vi "private-TestableClass FirstTest.vi"(8 "error in (no error)":errorcluster, 11 "Caraya-TestableClass in":refnum<class "Caraya-TestableClass.lvclass">) -> (0 "error out":errorcluster)   [LabVIEW 2013, in "Caraya-TestableClass.lvclass"]
uses:
  Caraya-TestableClass.lvclass
  Caraya-TestableClass.lvclass/Caraya-TestableClass.ctl
  classes/Test/Test.lvclass
  classes/Assert/Assert.lvclass
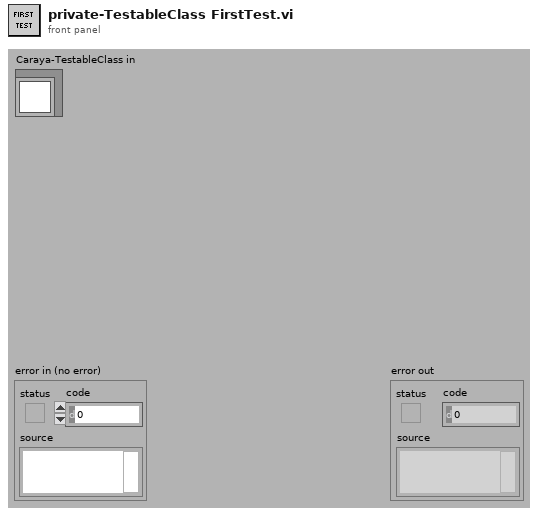
[diagram p1: front panel]
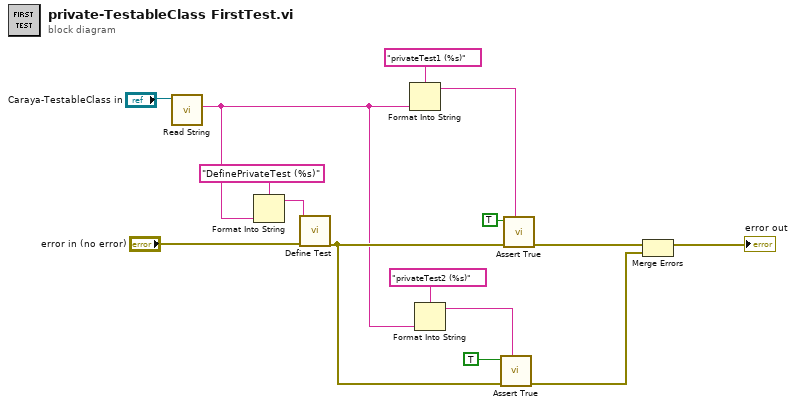
[diagram p0: block diagram]
diagram:
  n1 = call "Read String.vi"("Caraya-TestableClass in"="Caraya-TestableClass in") -> ("String"=w2:string)  [unwired: 9 in, 1 out]
  n2 = Format Into String(format string="DefinePrivateTest (%s)" ("Label (VI Title)"), w2) -> (resulting string=w8:string)  [unwired: 2 in, 1 out]
  n3 = call "Define Test.vi"("error in (no error)"="error in (no error)", "Label (VI Title)"=w8) -> ("error out"=w14:errorcluster)  [unwired: 9 in]
  n4 = Format Into String(format string="privateTest1 (%s)", w2) -> (resulting string=w4:string)  [unwired: 2 in, 1 out]
  n5 = Format Into String(format string="privateTest2 (%s)", w2) -> (resulting string=w1:string)  [unwired: 2 in, 1 out]
  n6 = call "Assert True.vi"("Label"=w1, "error in (no error)"=w14, "True?"=TRUE) -> ("error out"=w13:errorcluster)  [unwired: 8 in]
  n7 = call "Assert True.vi"("Label"=w4, "error in (no error)"=w14, "True?"=TRUE) -> ("error out"=w12:errorcluster)  [unwired: 8 in]
  n8 = Merge Errors(w12, w13) -> (→"error out":errorcluster)
